vi "Read Subpanel inside of.vi"(8 "error in (no error)":errorcluster, 11 "Fiber Auto Collimation panel in":refnum<class "Fiber Auto Collimation panel.lvclass">) -> (0 "error out":errorcluster, 2 "Subpanel inside of":refnum<vi>, 3 "Fiber Auto Collimation panel out":refnum<class "Fiber Auto Collimation panel.lvclass">)   [LabVIEW 2018, in "Fiber Auto Collimation panel.lvclass"]
doc: "The \"write\" accessor for this VI is set to Private because it should only be run by the \"Insert into subpanel\" VI.\n\nThis stores the reference to a sub-panel that this VI is currently running inside of. It's mostly needed to remove this VI when it finished running so a stopped VI isn't stuck in a subpanel."
uses:
  Fiber Auto Collimation panel.lvclass
  Fiber Auto Collimation panel.lvclass/Fiber Auto Collimation panel.ctl
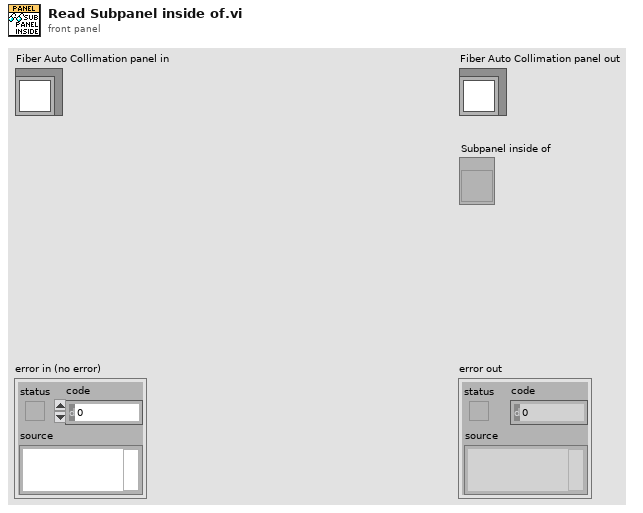
[diagram p1: front panel]
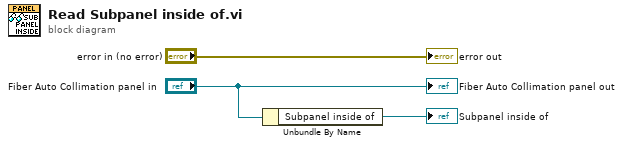
[diagram p0: block diagram]
diagram:
  n1 = Unbundle By Name("Fiber Auto Collimation panel in") -> ("Subpanel inside of"=→"Subpanel inside of":refnum<vi>)
  "error out" <- "error in (no error)"
  "Fiber Auto Collimation panel out" <- "Fiber Auto Collimation panel in"
